vi "GetFPGAPersonalityListInfo.vi"(7 "MetaDataObj in":refnum<class "MetaDataObj.lvclass">, 8 "error in (no error)":errorcluster, 10 "Project Title":string, 11 "ProdID":u32) -> (0 "error out":errorcluster, 1 "Available FPGA Tags":string[](array[string]), 2 "Available FPGA Personalities":string[](array[string]), 3 "Index for Default Personality":u16, 5 "MetaDataObj Out":refnum<class "MetaDataObj.lvclass">)   [LabVIEW 2021, in "myRIOMetaDataObj.lvclass"]
uses:
  myRIOMetaDataObj.lvclass
  <resource>/dialog/NewProjectWizard/MetaDataObj/MetaDataObj.lvclass
  <vilib>/Utility/error.llb/DialogType.ctl
  <vilib>/myRIO/Common/FPGA Personality Framework/Personality.lvlib
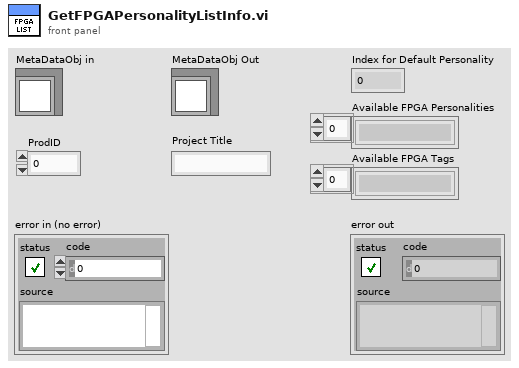
[diagram p1: front panel]
types:
  T1 = cluster{i32, "Property Value":string, "Property Value":string}
  T2 = cluster{i32, "Property Value":string, "Property Value":string}[]
  T3 = typedef "DialogType.ctl" = u16
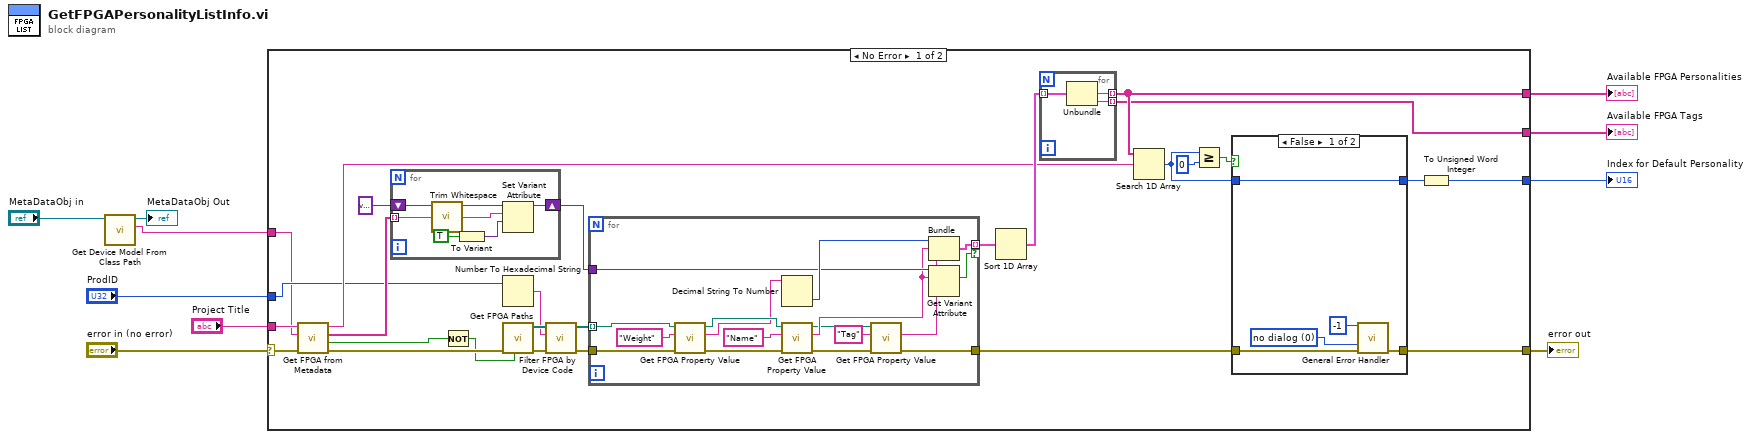
[diagram p0: block diagram]
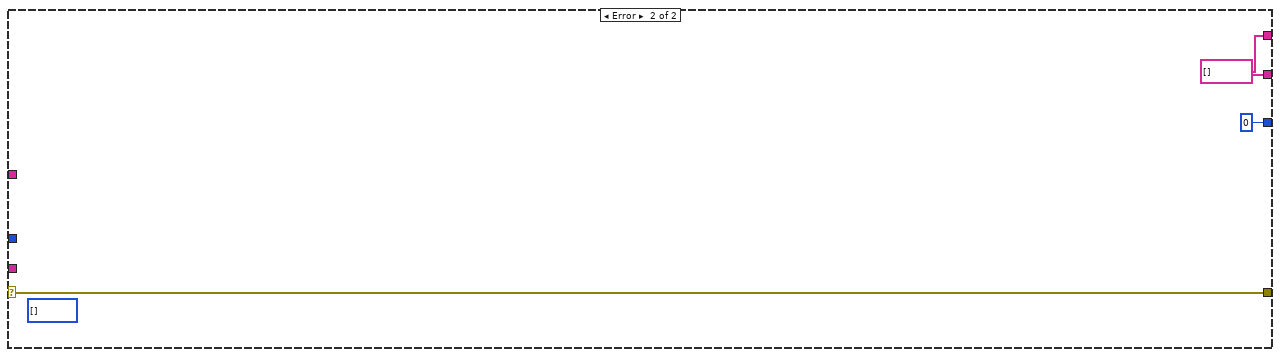
[diagram p3: hidden frame]
diagram:
  n1 = call "Get Device Model From Class Path.vi"("MetaDataObj in"="MetaDataObj in") -> ("Device Model Str"=w1:string, "MetaDataObj Out"=→"MetaDataObj Out":refnum<class "MetaDataObj.lvclass">)  [unwired: 8 in, 1 out]
  n2 = case shown="No Error" "error in (no error)" {
    selector: "error in (no error)" -> [w23 w73]
    tunnel: "ProdID" -> [w12 _]
    tunnel: "Project Title" -> [w32 _]
    tunnel: [w26 u16 0] -> w8
    tunnel: [w31 w71] -> w7
    tunnel: [w24 w73] -> w6
    tunnel: [w13 w71] -> w5
    tunnel: w1 -> [w11 _]
    frame No Error {
      n3 = call <vilib>:"Get FPGA from Metadata.vi"("error in (no error)"=w23, "Device Model Str"=w11, "Title"=w32) -> ("error out"=w22:errorcluster, "Customized?"=w18:bool, "Supported FPGA Personalities"=w16:string[], "Defaul FPGA Personality"=w33:string)  [unwired: 4 in, 1 out]
      n4 = for {
        tunnel: w16 -> [w41] mode=indexing
        shift-right: [w42] -> w14
        shift-left: variant -> [w43]
        n5 = call <vilib>:"Trim Whitespace.vi"("string"=w41) -> ("trimmed string"=w38:string)  [unwired: 1 in]
        n6 = To Variant(anything=TRUE) -> (Variant=w40:variant)
        n7 = Set Variant Attribute(Variant=w43, name=w38, value=w40) -> (Variant out=w42:variant)  [unwired: 1 in, 2 out]
      }
      n8 = Not(x=w18) -> (.not. x?=w17:bool)
      n9 = Number To Hexadecimal String(2:w12) -> (0:w30:string)  [unwired: 1 in]
      n10 = call <vilib>:"Get FPGA Paths.vi"("Filter Customized (T)"=w17, "error in (no error)"=w22) -> ("error out"=w36:errorcluster, "FPGA Personality File Paths"=w37:path[])  [unwired: 8 in]
      n11 = call <vilib>:"Filter FPGA by Device Code.vi"("error in (no error)"=w36, "Device Code"=w30, "FPGA Personality File Paths"=w37) -> ("error out"=w20:errorcluster, "Filtered FPGA Personality File Paths"=w35:path[])  [unwired: 7 in]
      n12 = for {
        tunnel: w35 -> [w67] mode=indexing
        tunnel: [w63] -> w21 mode=indexing if=w58
        tunnel: w20 -> [w62]
        tunnel: [w57] -> w19
        tunnel: w14 -> [w60]
        n13 = call <vilib>:"Get FPGA Property Value.vi"("error in (no error)"=w62, "Property Name"="Weight", "FPGA Personality File Path"=w67) -> ("error out"=w69:errorcluster, "Property Value"=w64:string, "Duplicated FPGA Personality File Path"=w66:path)  [unwired: 5 in, 1 out]
        n14 = Decimal String To Number(string=w64) -> (number=w65:i32)  [unwired: 2 in, 1 out]
        n15 = call <vilib>:"Get FPGA Property Value.vi"("error in (no error)"=w69, "Property Name"="Name", "FPGA Personality File Path"=w66) -> ("error out"=w61:errorcluster, "Property Value"=w59:string, "Duplicated FPGA Personality File Path"=w56:path)  [unwired: 5 in, 1 out]
        n16 = call <vilib>:"Get FPGA Property Value.vi"("error in (no error)"=w61, "Property Name"="Tag", "FPGA Personality File Path"=w56) -> ("error out"=w57:errorcluster, "Property Value"=w54:string)  [unwired: 5 in, 2 out]
        n17 = Bundle(w65, "Property Value"=w59, "Property Value"=w54) -> (w63:T1)  [unwired: 1 in]
        n18 = Get Variant Attribute(Variant=w60, name=w59) -> (found=w58:bool)  [unwired: 2 in, 3 out]
      }
      n19 = Sort 1D Array(array=w21) -> (sorted array=w34:T2)
      n20 = for {
        tunnel: w34 -> [w53] mode=indexing
        tunnel: [w52] -> w31 mode=indexing
        tunnel: [w51] -> w13 mode=indexing
        n21 = Unbundle(w53) -> ("Property Value"=w52:string, "Property Value"=w51:string)  [unwired: 1 out]
      }
      n22 = Search 1D Array(1D array=w31, element=w33) -> (index of element=w29:i32)  [unwired: 1 in]
      n23 = Greater Or Equal?(x=w29, y=0) -> (x >= y?=w27:bool)
      n24 = case shown="False" w27 {
        tunnel: w29 -> [w48 w50]
        tunnel: [w48 w50] -> w25
        tunnel: w19 -> [w47 w49]
        tunnel: [w45 w49] -> w24
        frame False {
          w46 = T3 0 items=["no dialog", "OK message", "continue or stop message", "OK message + warnings", "continue/stop + warnings"] ("type of dialog (OK msg:1)")
          n25 = call <vilib>:"General Error Handler.vi"("[error code] (0)"=-1, "type of dialog (OK msg:1)"=w46, "error in (no error)"=w47) -> ("error out"=w45:errorcluster)  [unwired: 8 in, 4 out]
        }
        frame True {
        }
      }
      n26 = To Unsigned Word Integer(number=w25) -> (unsigned 16bit integer=w26:u16)
    }
    frame Error {
      (unwired) i32[] []
      w71 = string[] []
    }
  }
  "Available FPGA Personalities" <- w7
  "Index for Default Personality" <- w8
  "error out" <- w6
  "Available FPGA Tags" <- w5
